vi "FRCts20_Backend_Comment_POST_reform.vi"(7 "Notes":T1, 8 "error in (no error)":errorcluster, 11 "recordset data":variant[][](array[variant])) -> (0 "error out":errorcluster, 3 "data string":string)   [LabVIEW 2014, in "FRCts20_Backend_Engine.lvlib"]
doc: "Returns whether a new comment was created & the new comment's note index"
uses:
  FRCts20_Backend_Engine.lvlib
  FRCts20_Backend_API/Notes.ctl
  FRCts20_Backend_API/ApiReturn.ctl
  FRCts20_Backend_API/NotesRoot.ctl
  <vilib>/addons/database/_DB Variant To Data/Database Variant To Data.xnode
  FRCts20_Backend_API/FRCts20_Backend_API.lvlib
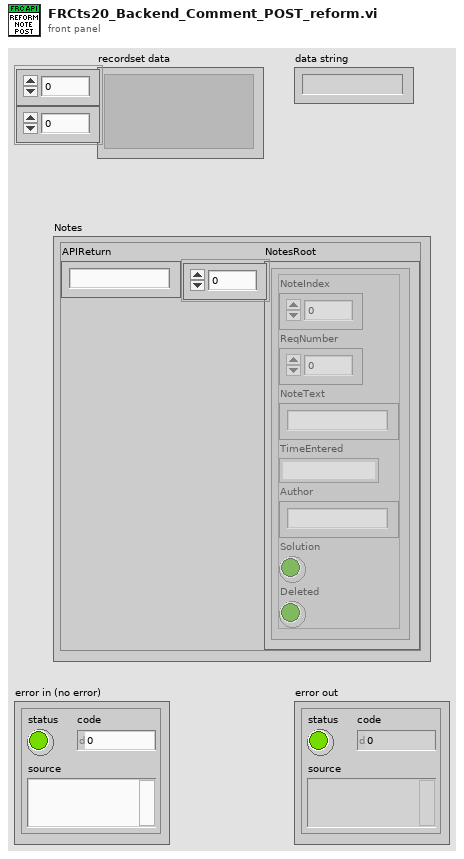
[diagram p1: front panel]
types:
  T1 = typedef "FRCts20_Backend_Engine.lvlib/FRCts20_Backend_API.lvlib/Notes.ctl" = cluster{"APIReturn":T2, "NotesRoot":T3}
  T2 = typedef "FRCts20_Backend_Engine.lvlib/FRCts20_Backend_API.lvlib/ApiReturn.ctl" = string
  T3 = typedef "FRCts20_Backend_Engine.lvlib/FRCts20_Backend_API.lvlib/NotesRoot.ctl" = cluster{"NoteIndex":u32, "ReqNumber":i32, "NoteText":string, "TimeEntered":string, "Author":string, "Solution":bool, "Deleted":bool}[]
  T4 = cluster{"NoteIndex":u32, "ReqNumber":i32, "NoteText":string, "TimeEntered":string, "Author":string, "Solution":bool, "Deleted":bool}
  T5 = cluster{"NoteIndex":u32, "ReqNumber":i32, "NoteText":string, "TimeEntered":string, "Author":string, "Solution":bool, "Deleted":bool}[]
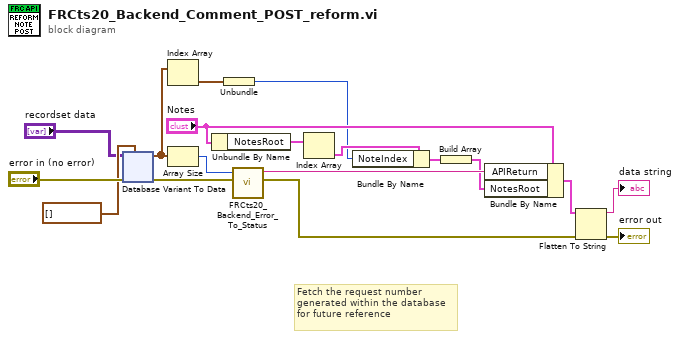
[diagram p0: block diagram]
diagram:
  # "Fetch the request number\ngenerated within the database\nfor future reference"
  n1 = xnode "Database Variant To Data"("database variant"="recordset data", "error in"="error in (no error)", "type"=cluster{u32}[] []) -> ("data"=w8:cluster{u32}[], "error out"=w15:errorcluster)
  n2 = Index Array(array=w8) -> (element=w11:cluster{u32})  [unwired: 1 in]
  n3 = Array Size(array=w8) -> (size(s)=w7:i32)
  n4 = Unbundle By Name("Notes") -> ("NotesRoot"=w5:T3)
  n5 = Unbundle(w11) -> (w3:u32)
  n6 = call "FRCts20_Backend_Error_To_Status.vi"("error in (no error)"=w15, "rows affected"=w7) -> ("error out"=w14:errorcluster, "String"=w16:string)  [unwired: 8 in]
  n7 = Index Array(array=w5) -> (element=w4:T4)  [unwired: 1 in]
  n8 = Bundle By Name(cluster=w4, "NoteIndex"=w3) -> (w2:T4)
  n9 = Build Array(w2) -> (w1:T5)
  n10 = Bundle By Name(cluster="Notes", "APIReturn"=w16, "NotesRoot"=w1) -> (w12:T1)
  n11 = Flatten To String(anything=w12, error in (no error)=w14) -> (data string=→"data string":string, error out=→"error out":errorcluster)  [unwired: 2 in, 1 out]
